vi "finishABCPassPlay.vi"(8 "error in (no error)":errorcluster, 10 "Game in":refnum<class "Game.lvclass">, 11 "ABCPassPlay in":refnum<class "ABCPassPlay.lvclass">) -> (0 "error out":errorcluster, 2 "Boolean":bool, 3 "ABCPassPlay out":refnum<class "ABCPassPlay.lvclass">)   [LabVIEW 2021, in "ABCPassPlay.lvclass"]
uses:
  ABCPassPlay.lvclass
  D:/RoboIme/horie/SSL_AI/Play_class/Play.lvclass
  Game_class/Game.lvclass
  Referee_class/command_interpreted.ctl
  Game_class/Game.lvclass/Game.ctl
  Events_class/Events.lvclass/Events.ctl
  Ball_class/Ball.lvclass/Ball.ctl
  Referee_class/Referee.lvclass/Referee.ctl
  Team_class/Team.lvclass/Team.ctl
  Game_class/Read Referee.vi
  Referee_class/Read command_interpreted.vi
  Game_class/Read EventsRef.vi
  Game_class/Read BallRef.vi
  Game_class/Read OffensiveTeam.vi
  Team_class/Read RobotRef.vi
  Ball_class/Read z.vi
  Events_class/Read touch.vi
  Events_class/Read id_touch.vi
  Events_class/Read ball_out.vi
  Ally_class/Ally.lvclass
  D:/RoboIme/horie/SSL_AI/Team_class/Team.lvclass
  Events_class/Events.lvclass
  Ball_class/Ball.lvclass
  Robot_class/Robot.lvclass
  Referee_class/Referee.lvclass
  Play_class/Play.lvclass
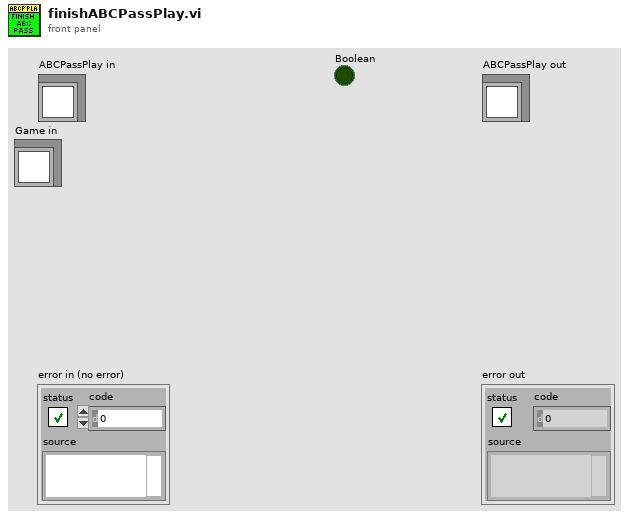
[diagram p1: front panel]
types:
  T1 = typedef "command_interpreted.ctl" = enum16{"Goal Ally", "Goal Enemy", "Ball Placement Enemy", "Ball Placement Ally", "Normal Half Time", "Extra Time  Break", "Extra Half Time", "None", "Post Game", "PKA Normal Start", "Prepare Kickoff Ally", "PKE Normal Start", "Prepare Kickoff Enemy", "Force Start", "Halt", "Timeout", "Prepare Penalty Ally", "Prepare Penalty Enemy", "PPA NormalStart", "PPE Normal Start", "Indirect Free Ally", "Direct Free Enemy", "Direct Free Ally", "Indirect Free Enemy", "Stop"}
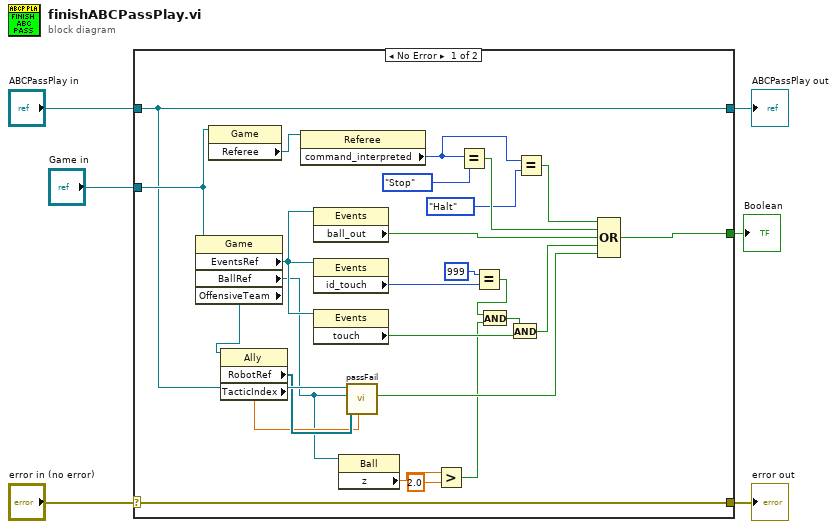
[diagram p0: block diagram]
diagram:
  n1 = case shown="No Error" "error in (no error)" {
    selector: "error in (no error)" -> [w32 w34]
    tunnel: [w32 w34] -> w5
    tunnel: [w17 w33] -> w3
    tunnel: "ABCPassPlay in" -> [w17 w33]
    tunnel: "Game in" -> [w19 _]
    tunnel: [w18 _] -> w1
    frame No Error {
      n2 = property class="Game"(reference=w19) -> ("EventsRef"=w31:refnum<class "Events.lvclass">, "BallRef"=w12:refnum<class "Ball.lvclass">, "OffensiveTeam"=w16:refnum<class "Ally.lvclass">)  [unwired: 1 in, 2 out]
      n3 = property class="Game"(reference=w19) -> ("Referee"=w26:refnum<class "Referee.lvclass">)  [unwired: 1 in, 2 out]
      n4 = property class="Ally"(reference=w16) -> ("RobotRef"=w15:refnum<class "Robot.lvclass">[], "TacticIndex"=w13:dbl)  [unwired: 1 in, 2 out]
      n5 = property class="Referee"(reference=w26) -> ("command_interpreted"=w22:T1)  [unwired: 1 in, 2 out]
      n6 = property class="Events"(reference=w31) -> ("ball_out"=w28:bool)  [unwired: 1 in, 2 out]
      n7 = property class="Events"(reference=w31) -> ("id_touch"=w29:i32)  [unwired: 1 in, 2 out]
      n8 = property class="Events"(reference=w31) -> ("touch"=w25:bool)  [unwired: 1 in, 2 out]
      n9 = property class="Ball"(reference=w12) -> ("z"=w11:dbl)  [unwired: 1 in, 2 out]
      n10 = call "passFail.vi"("TacticIndex"=w13, "Offensive Robots"=w15, "Ball"=w12, "Play in"=w17) -> ("PassFail?"=w14:bool)  [unwired: 5 in, 2 out]
      n11 = Greater?(x=w11, y=2.0) -> (0:w8:bool)
      n12 = Equal?(x=w22, y=command_interpreted."Stop") -> (x = y?=w23:bool)
      n13 = Equal?(x=999 ("id_touch"), y=w29) -> (x = y?=w9:bool)
      n14 = And(x=w9, y=w8) -> (x .and. y?=w7:bool)
      n15 = And(x=w7, y=w25) -> (x .and. y?=w27:bool)
      n16 = Equal?(x=w22, y=command_interpreted."Halt") -> (x = y?=w20:bool)
      n17 = Compound Arithmetic op=OR(w20, w23, w28, w27, w14) -> (w18:bool)
    }
    frame Error {
    }
  }
  "error out" <- w5
  "ABCPassPlay out" <- w3
  "Boolean" <- w1
